vi "Autonomous Independent.vi"() -> ()   [LabVIEW 2014]
doc: "This VI is called when autonomous begins, and will automatically be terminated when autonomous ends. You can carry out timed or sensor driven robot movement independently without needing to return to the caller."
uses:
  <vilib>/Rock Robotics/WPI/RobotDrive/WPI_RobotDriveMecanumDrive_Cartesian.vi
  <vilib>/Rock Robotics/WPI/Solenoid/WPI_SolenoidValue.ctl
  Robot Global Data.vi
  <vilib>/Rock Robotics/WPI/Solenoid/WPI_SolenoidSetEnum.vi
  <vilib>/Rock Robotics/WPI/SafetyOutput/WPI_SafetyOutputConfigMenu.ctl
  navx-mxp_NEW/roborio/labview/navX-MXP Library/navX-MXP IMU.lvlib
  <vilib>/Rock Robotics/Network Tables/SD Read Boolean.vi
  <vilib>/Rock Robotics/Network Tables/SD Read String.vi
  <vilib>/Rock Robotics/Network Tables/SD Write Numeric Array.vi
  <vilib>/Rock Robotics/WPI/RobotDrive/WPI_RobotDriveMecanumDrive_Polar.vi
panel:
  out "MODE: AUTO ZONE":bool
  out "MODE: HPS":bool
  out "AUTO?":bool
  # "EDITED: 3/2/15"
  # "Be sure to right-click and choose Data Operations>>Make Current Value default if you want to save the array values with the VI"
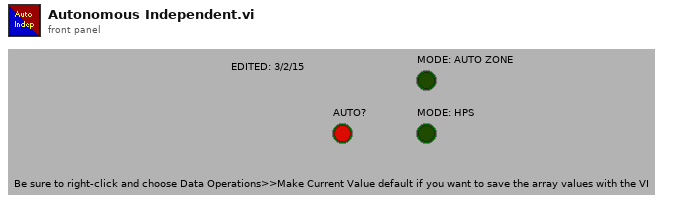
[diagram p1: front panel]
types:
  T1 = typedef "WPI_JoystickDevRef.ctl" = cluster{"Device":T2}
  T2 = typedef "WPI_JoystickDeviceEnum.ctl" = enum16{"USB 0", "USB 1", "USB 2", "USB 3", "USB 4", "USB 5"}
  T3 = typedef "WPI_SafetyOutputConfigMenu.ctl" = enum16{"Enable", "Disable"}
  T4 = typedef "WPI_SolenoidValue.ctl" = enum16{"Off", "On", "Forward", "Reverse"}
  T5 = typedef "navX-MXP IMU.lvlib/navX Device TypeDef.ctl" = cluster{"navX Interface Protocol":T6, "navX Interface Protocol TypeDefs":cluster{"SPIDevRef":T7, "I2CDevRef":T10}, "navX System Information":cluster{"Board Information":T12, "Status":T13, "Offsets":T17}, "navX Common Information":cluster{"Update Rate (4Hz-60Hz)":T18, "refnum name":string, "error":errorcluster}}
  T6 = typedef "navX-MXP IMU.lvlib/navX Interface Protocol.ctl" = enum16{"SPI", "I2C"}
  T7 = typedef "WPI_SPIDevRef.ctl" = cluster{"DevStatus":errorcluster, "Handle":i32, "Controller":T8, "SPI Bus":T9}
  T8 = typedef "FPGA_TypedefDigitalModule.ctl" = enum16{"Controller 1"}
  T9 = typedef "spi_bus.ctl" = enum16{"SPI On-Board, CS0", "SPI On-Board, CS1", "SPI On-Board, CS2", "SPI On-Board, CS3", "SPI MXP", "Invalid"}
  T10 = typedef "WPI_I2CDevRef.ctl" = cluster{"DevStatus":errorcluster, "Controller":T8, "Device Address":u8, "Handle":i32, "I2C Bus":T11}
  T11 = typedef "i2c_bus.ctl" = enum16{"I2C On-Board", "I2C MXP", "Invalid"}
  T12 = typedef "navX-MXP IMU.lvlib/navX Board Information.ctl" = cluster{"WhoAmI (50 | 0x32)":u8, "Board Revision":u8, "Firmware Major Version":u8, "Firmware Minor Version":u8}
  T13 = typedef "navX-MXP IMU.lvlib/navX Status Data.ctl" = cluster{"Update Rate Hz":u8, "Accelerometer Full-Scale Range":u8, "Gyro Full-Scale Range":u16, "NAVX_OP_STATUS":T14, "NAVX_CAL_STATUS":T15, "NAVX_SELFTEST_STATUS":u8, "NAVX_SENSOR_STATUS":T16}
  T14 = typedef "navX-MXP IMU.lvlib/navX NAVX_OP_STATUS.ctl" = u8
  T15 = typedef "navX-MXP IMU.lvlib/navX NAVX_CAL_STATUS.ctl" = u8
  T16 = typedef "navX-MXP IMU.lvlib/navX NAVX_SENSOR_STATUS.ctl" = cluster{"MOVING":bool, "YAW_STABLE":bool, "MAG_DISTURBANCE":bool, "ALTITUDE_VALID":bool, "SEALEVEL_PRESS_SET":bool, "FUSED_HEADING_VALID":bool}
  T17 = typedef "navX-MXP IMU.lvlib/navX Offsets Data.ctl" = cluster{"Yaw":dbl, "Quat W":dbl, "Quat X":dbl, "Quat Y":dbl, "Quat Z":dbl}
  T18 = typedef "navX-MXP IMU.lvlib/navX Update Rate.ctl" = u8
  T19 = cluster{"proportional gain (Kc)":dbl, "integral time (Ti, min)":dbl, "derivative time (Td, min)":dbl}
  T20 = typedef "WPI_RobotDriveDevRef.ctl" = cluster{"DevStatus":errorcluster, "Motors[]":T21[], "Square Inputs":bool, "Max Output":dbl}
  T21 = typedef "WPI_MotorControlDeviceRef.ctl" = cluster{"DeviceStatus":errorcluster, "Type":T22, "PWM":cluster{"Controller":T8, "PWM Channel":T23, "DeadBand":T24}, "CAN":cluster{"Device Number":u8, "Control Mode":T25, "Semaphore":T26, "Max Vout":dbl, "TalonSRX Control Mode":T27}, "Invert":bool, "TransformRef":T28, "InvTransformRef":T28}
  T22 = typedef "WPI_MotorControlType.ctl" = enum16{"PWM", "CAN", "CANTalonSRX"}
  T23 = typedef "FPGA_DIOPWMChannel.ctl" = enum8{"PWM 0", "PWM 1", "PWM 2", "PWM 3", "PWM 4", "PWM 5", "PWM 6", "PWM 7", "PWM 8", "PWM 9", "PWM MXP 0", "PWM MXP 1", "PWM MXP 2", "PWM MXP 3", "PWM MXP 4", "PWM MXP 5", "PWM MXP 6", "PWM MXP 7", "PWM MXP 8", "PWM MXP 9", "Invalid"}
  T24 = typedef "WPI_PWMDeadband.ctl" = cluster{"Name":string, "maxPositivePwm":i32, "minPositivePwm":i32, "centerPwm":i32, "maxNegativePwm":i32, "minNegativePwm":i32, "angularRange":u16}
  T25 = typedef "WPI_CANJaguar_ControlMode.ctl" = enum8{"Percent VBus", "Current", "Speed", "Position", "Voltage"}
  T26 = typedef "Semaphore RefNum" = refnum<k1>
  T27 = typedef "WPI_CANTalonSRX_APIControlMode.ctl" = enum8{"Percent VBus", "Speed", "Position", "Slave", "Unchanged / Invalid"}
  T28 = typedef "WPI_PWMTransform_ConPane.ctl" = refnum<vi>
  T29 = typedef "WPI_SolenoidDevRef.ctl" = cluster{"DevStatus":errorcluster, "Pneumatics Control Module":u8, "Forward Solenoid Channel":T30, "Reverse Solenoid Channel":T30}
  T30 = typedef "WPI_SolenoidChannel.ctl" = enum8{"Solenoid 0", "Solenoid 1", "Solenoid 2", "Solenoid 3", "Solenoid 4", "Solenoid 5", "Solenoid 6", "Solenoid 7", "Invalid"}
  T31 = typedef "WPI_DigitalInputDevRef.ctl" = cluster{"DevStatus":errorcluster, "DIO Channel":T32, "Controller":T8}
  T32 = typedef "FPGA_DIOChannel.ctl" = enum8{"DIO 0", "DIO 1", "DIO 2", "DIO 3", "DIO 4", "DIO 5", "DIO 6", "DIO 7", "DIO 8", "DIO 9", "DIO MXP 0", "DIO MXP 1", "DIO MXP 2", "DIO MXP 3", "DIO MXP 4", "DIO MXP 5", "DIO MXP 6", "DIO MXP 7", "DIO MXP 8", "DIO MXP 9", "DIO MXP 10", "DIO MXP 11", "DIO MXP 12", "DIO MXP 13", "DIO MXP 14", "DIO MXP 15", "Invalid"}
  T33 = cluster{"PID":dbl, "integral time (Ti, min)":dbl, "derivative time (Td, min)":dbl}
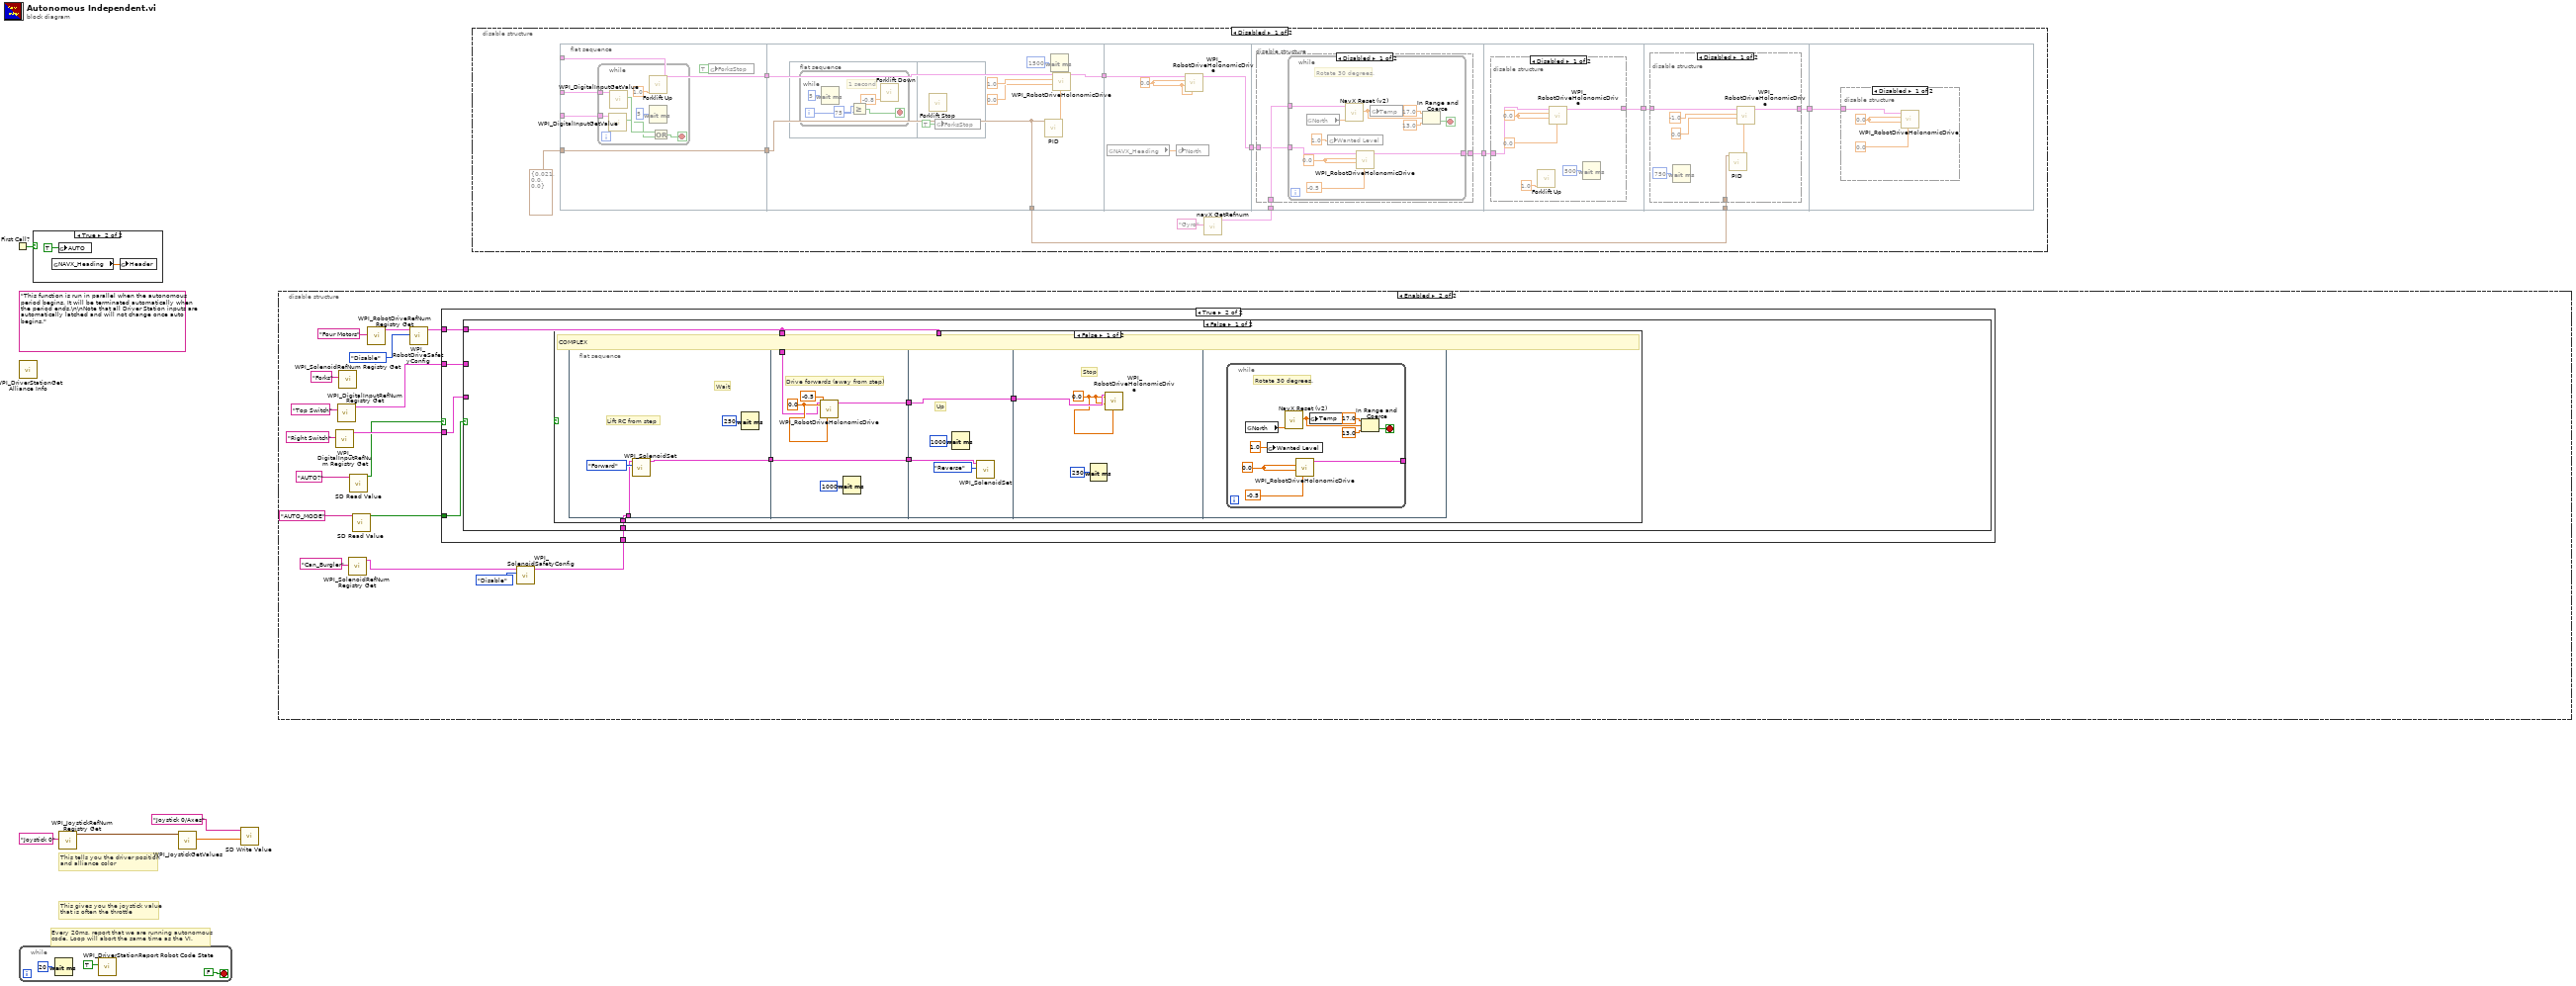
[diagram p0: block diagram]
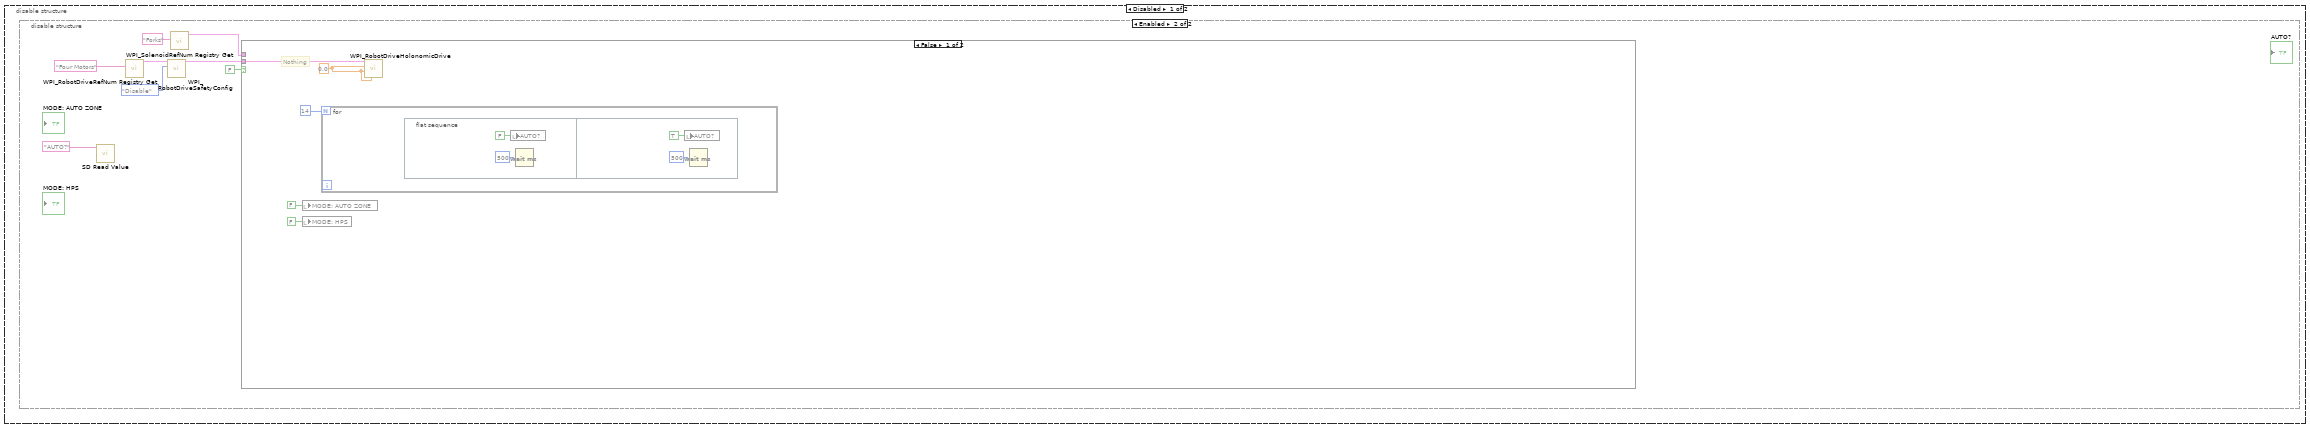
[diagram p7: hidden frame]
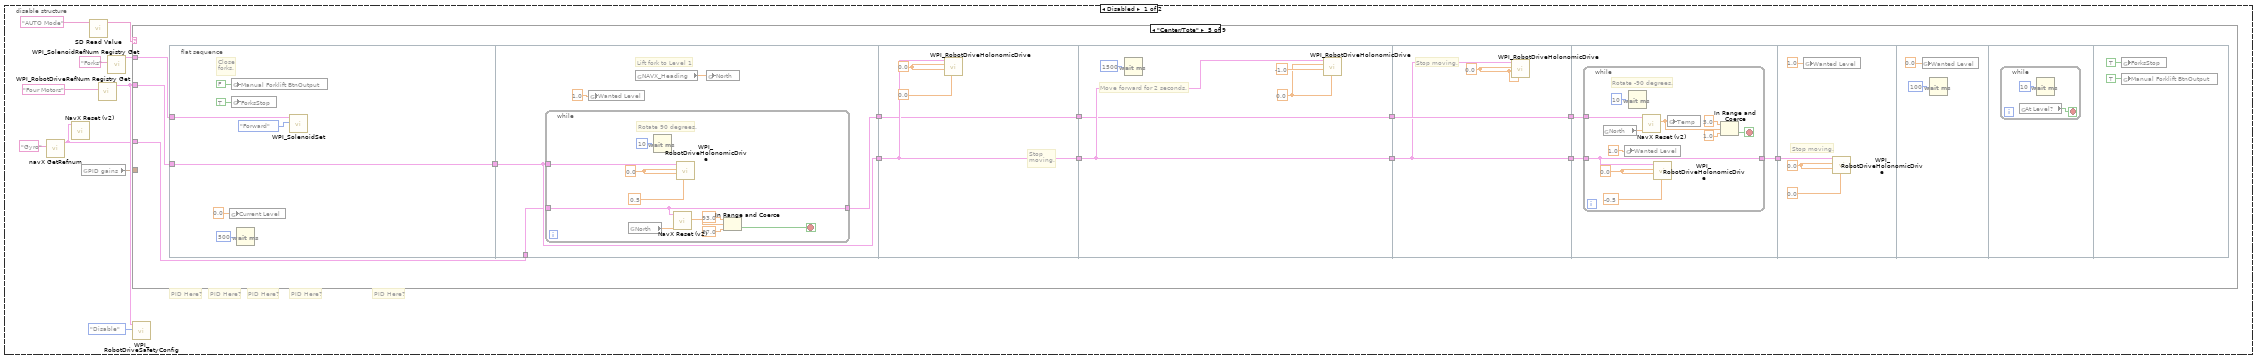
[diagram p8: hidden frame]
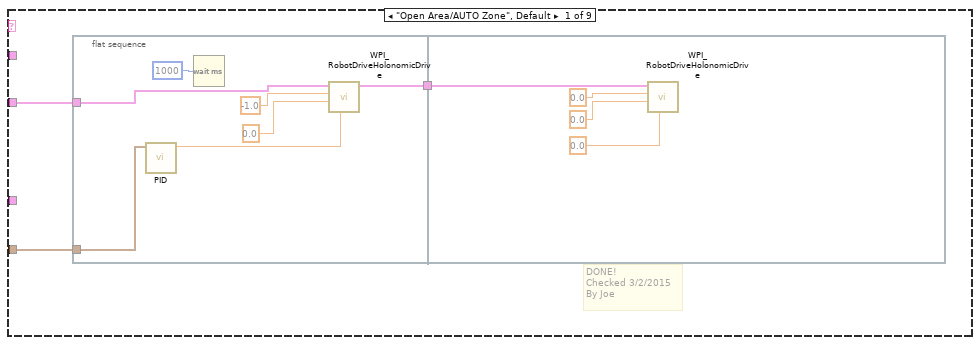
[diagram p9: hidden frame]
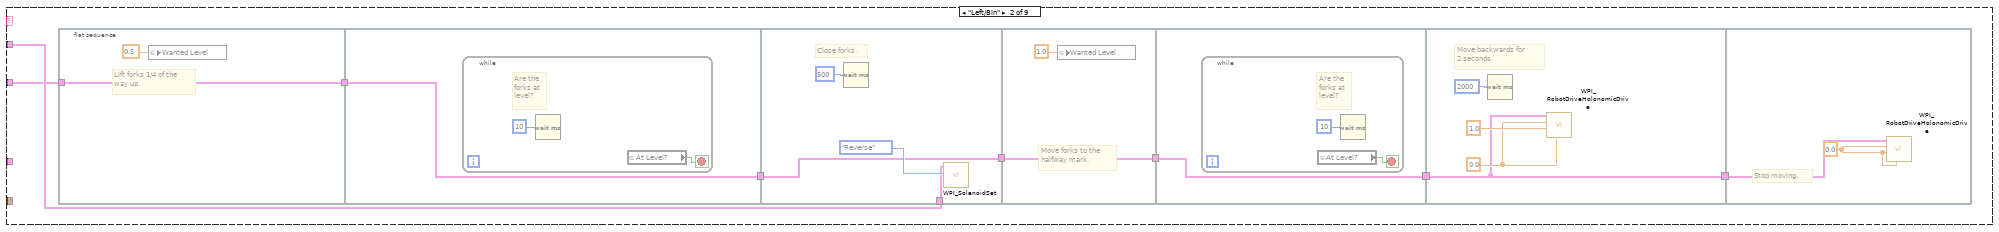
[diagram p10: hidden frame]
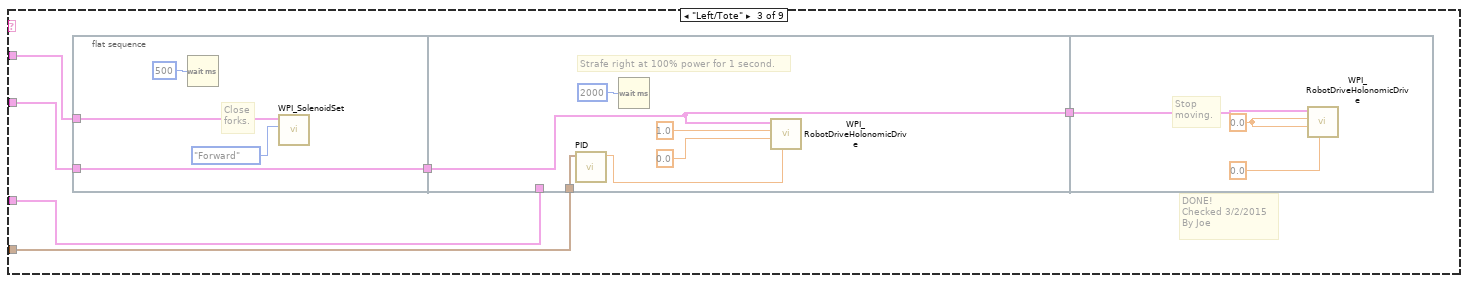
[diagram p11: hidden frame]
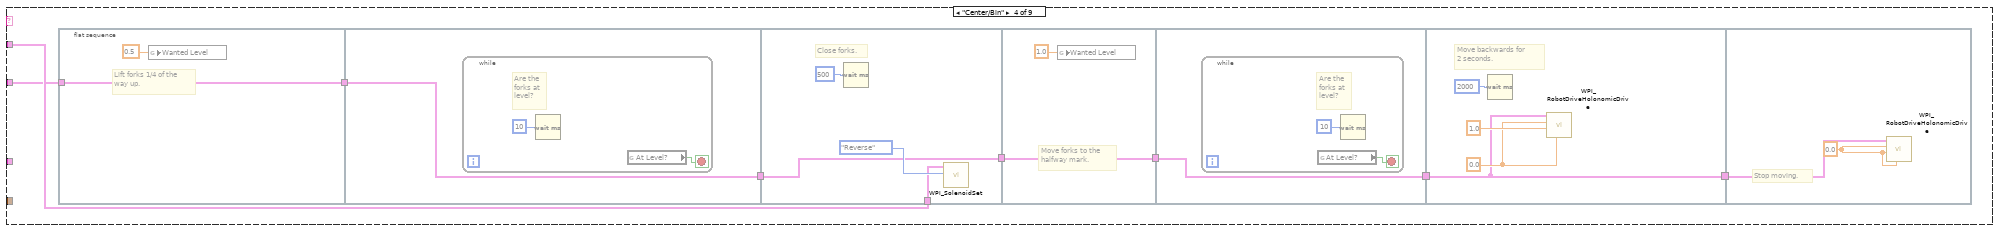
[diagram p12: hidden frame]
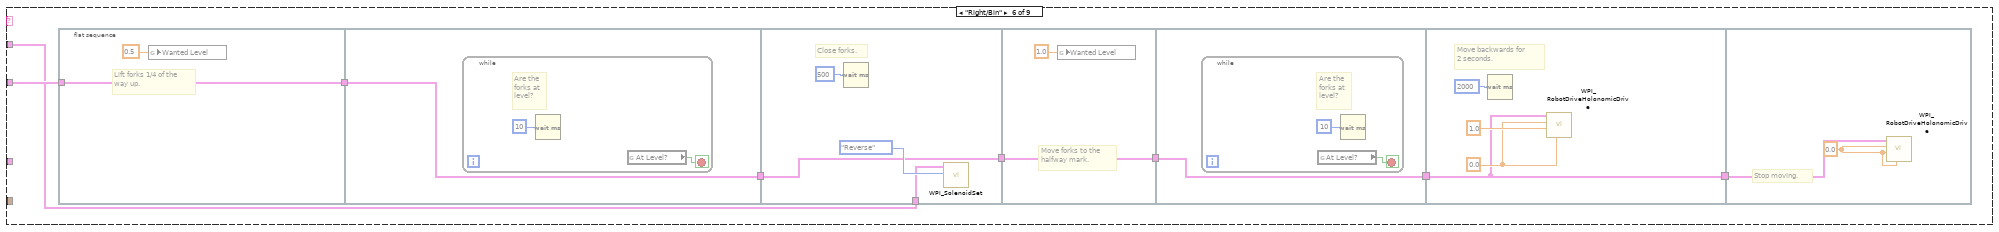
[diagram p13: hidden frame]
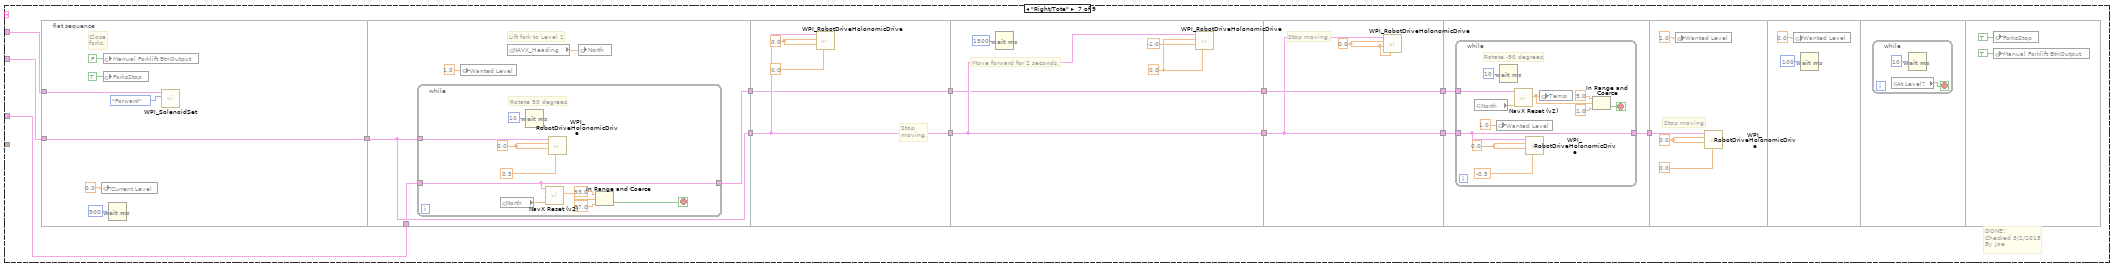
[diagram p14: hidden frame]
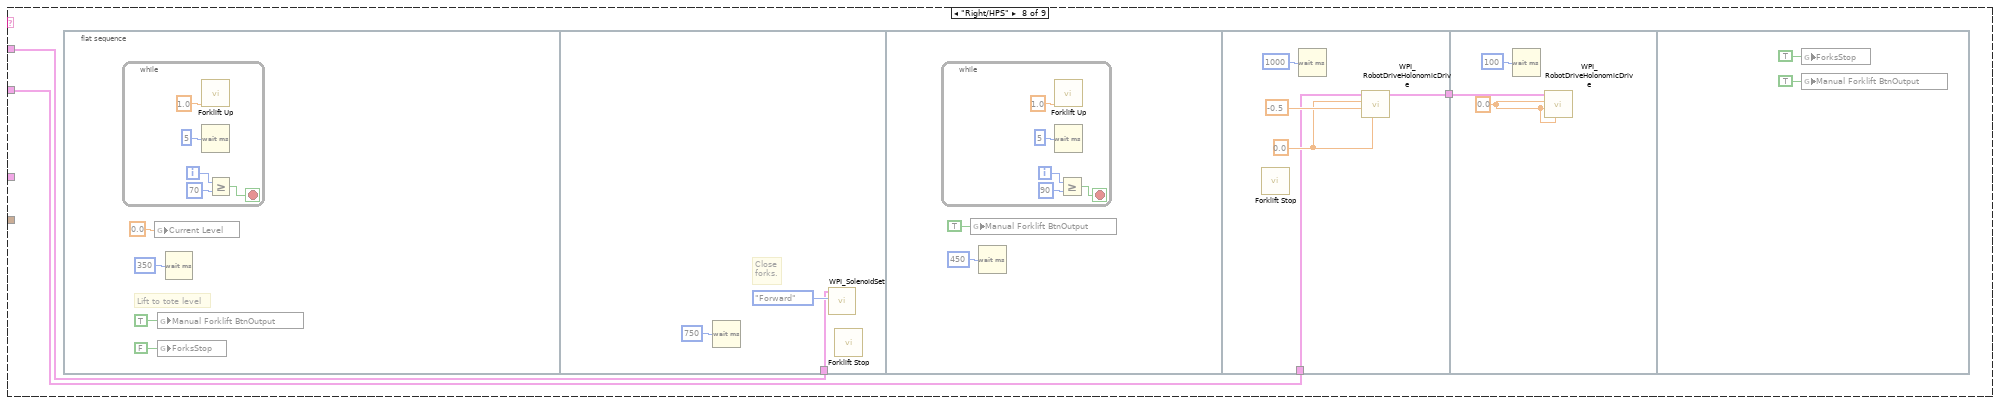
[diagram p15: hidden frame]
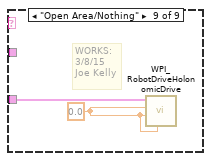
[diagram p16: hidden frame]
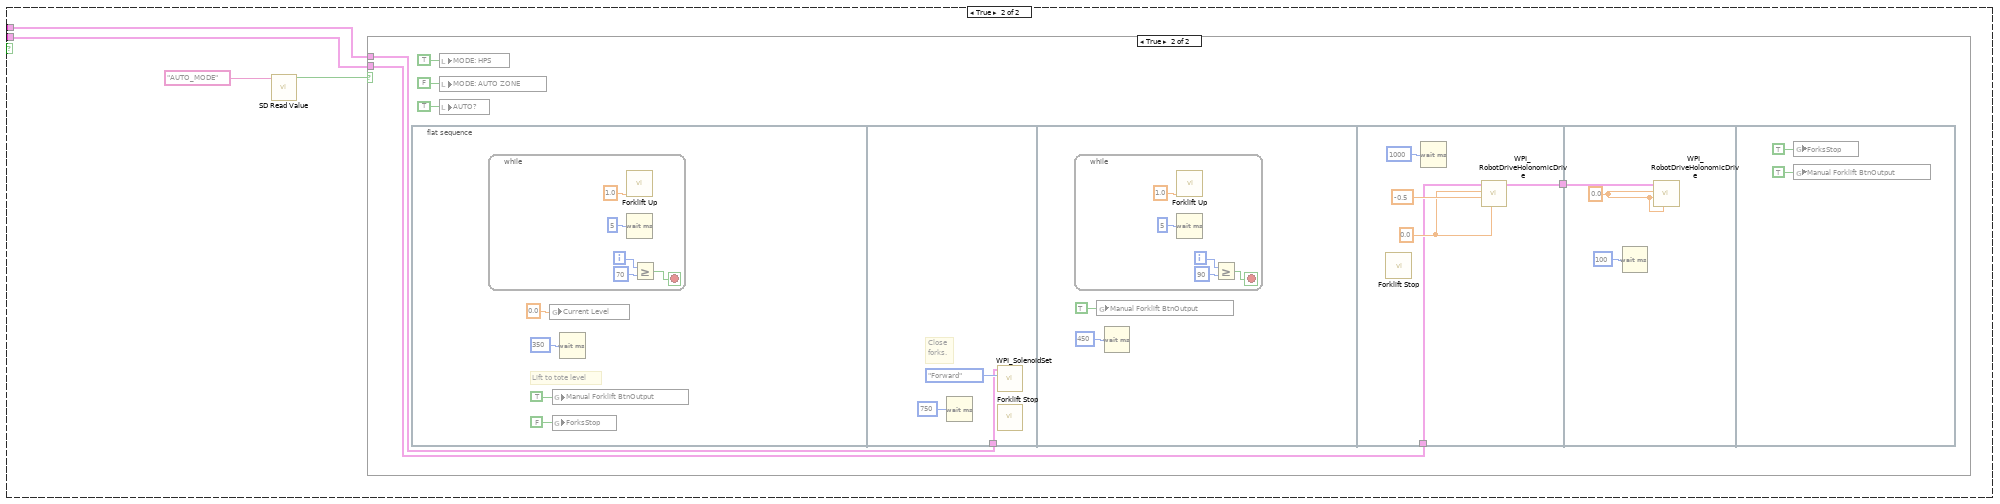
[diagram p17: hidden frame]
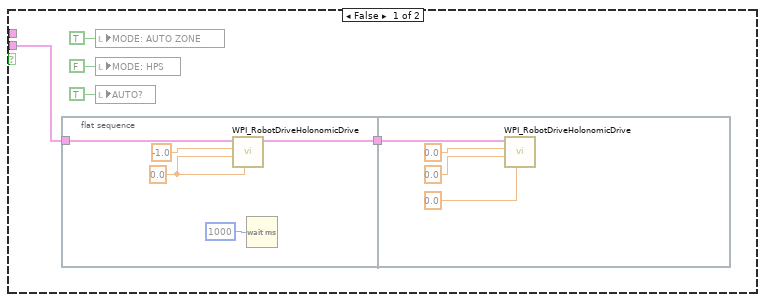
[diagram p18: hidden frame]
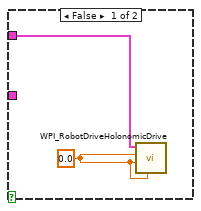
[diagram p19: hidden frame]
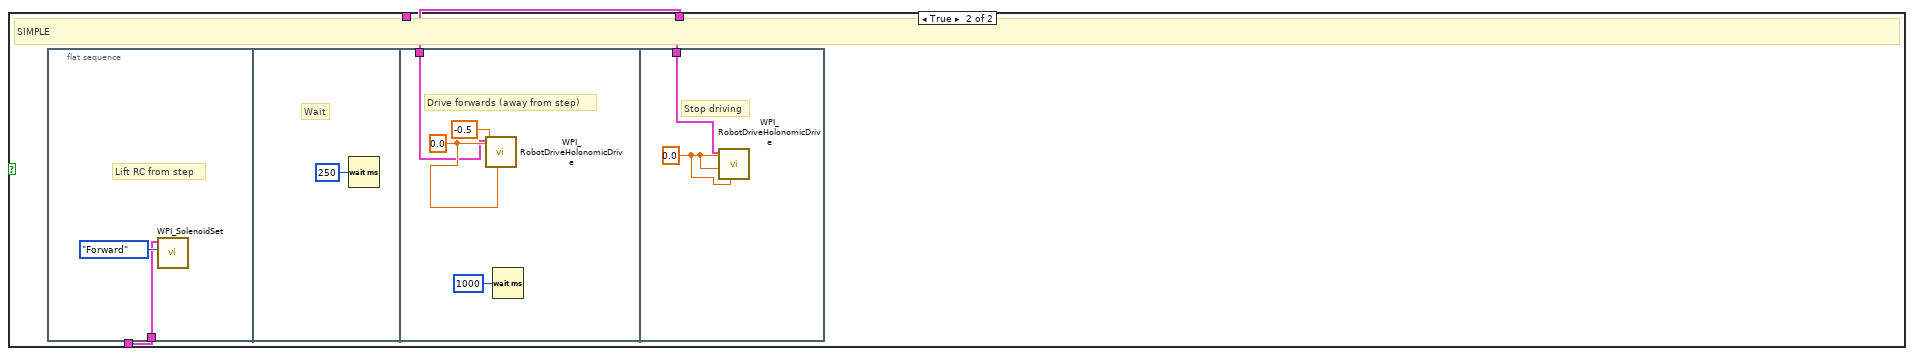
[diagram p20: hidden frame]
diagram:
  (unwired) "This function is run in parallel when the autonomous period begins. It will be terminated automatically when the period ends.\n\nNote that all Driver Station inputs are automatically latched and will not change once auto begins."
  # "Every 20ms, report that we are running autonomous\ncode. Loop will abort the same time as the VI."
  # "This gives you the joystick value\nthat is often the throttle"
  # "This tells you the driver position\nand alliance color"
  n1 = First Call?() -> (First Call?: T/F=w1:bool)
  n2 = call <vilib>:"WPI_DriverStationGet Alliance Info.vi"() -> ()  [unwired: 12 out]
  n3 = while {
    stop <- FALSE stop-if-true
    n4 = Wait (ms)(milliseconds to wait=u32 20) -> ()  [unwired: 1 out]
    n5 = call <vilib>:"WPI_DriverStationReport Robot Code State.vi"("Autonomous"=TRUE) -> ()  [unwired: 10 in, 1 out]
  }
  n6 = case shown="True" w1 {
    frame False {
    }
    frame True {
      n7 = global read "Robot Global Data.vi" "NAVX_Heading"() -> (w10:dbl)
      n8 = global write "Robot Global Data.vi" "AUTO"(TRUE ("AUTO")) -> ()
      n9 = global write "Robot Global Data.vi" "Header"(w10) -> ()
    }
  }
  n10 = call <vilib>:"WPI_JoystickRefNum Registry Get.vi"("refnum name"="Joystick 0") -> ("JoystickDevRef"=w4:T1)  [unwired: 1 in, 9 out]
  n11 = call <vilib>:"WPI_JoystickGetValues.vi"("JoystickDevRef"=w4) -> ("Axes"=w2:dbl[])  [unwired: 6 in, 4 out]
  n12 = call-poly <vilib>:"SD Write Value.vi"("Numeric Array"=w2, "Name"="Joystick 0/Axes") -> ()  [unwired: 8 in, 2 out]
  n13 = disable-structure shown="Enabled" {
    frame Disabled {
      n14 = disable-structure shown="Enabled" {
        frame Disabled {
          # "PID Here?"
          # "PID Here?"
          # "PID Here?"
          # "PID Here?"
          # "PID Here?"
          n15 = call "navX GetRefnum.vi"("refnum name"="Gyro") -> ("navX Device TypeDef"=w13:T5)  [unwired: 9 in, 1 out]
          n16 = call "NavX Reset (v2).vi"("navX Device TypeDef"=w13) -> ()  [unwired: 10 in, 1 out]
          n17 = global read "Robot Global Data.vi" "PID gains"() -> (w12:T19)
          n18 = call-poly <vilib>:"SD Read Value.vi"("Name"="AUTO Mode") -> ("String"=w20:string)  [unwired: 8 in, 2 out]
          n19 = call <vilib>:"WPI_RobotDriveRefNum Registry Get.vi"("refnum name"="Four Motors") -> ("RobotDriveDevRef"=w16:T20)  [unwired: 9 in, 1 out]
          n20 = call <vilib>:"WPI_SolenoidRefNum Registry Get.vi"("refnum name"="Forks") -> ("SolenoidDevRef"=w17:T29)  [unwired: 9 in, 1 out]
          n21 = case shown="\"Center/Tote\"" w20 {
            tunnel: w16 -> [w23 w41 w67 w86 w112 w186 w218 w281 w312]
            tunnel: w17 -> [_ w42 w68 w87 w111 w185 w217 w282 _]
            tunnel: w13 -> [_ _ w65 _ w110 _ w215 _ _]
            tunnel: w12 -> [w21 _ w63 _ _ _ _ _ _]
            frame "Open Area/AUTO Zone", Default {
              # "DONE!\nChecked 3/2/2015\nBy Joe"
              n22 = flat-sequence {
                tunnel: w23 -> [w27]
                tunnel: [w26] -> w22
                tunnel: w21 -> [w24]
                tunnel: w22 -> [w31]
                frame #0 {
                  n23 = call "PID.vi"("PID gains"=w24) -> ("output"=w25:dbl)  [unwired: 10 in]
                  n24 = Wait (ms)(milliseconds to wait=u32 1000) -> ()  [unwired: 1 out]
                  n25 = call-poly <vilib>:"WPI_RobotDriveHolonomicDrive.vi"("Rotation"=w25, "Y"=0.0, "X"=-1.0, "RobotDriveDevRef"=w27) -> ("RobotDriveDevRef"=w26:T20)  [unwired: 5 in, 2 out]
                }
                frame #1 {
                  n26 = call-poly <vilib>:"WPI_RobotDriveHolonomicDrive.vi"("Rotation"=0.0, "Y"=0.0, "X"=0.0, "RobotDriveDevRef"=w31) -> ()  [unwired: 5 in, 3 out]
                }
              }
            }
            frame "Left/Bin" {
              n27 = flat-sequence {
                tunnel: [w43] -> w38
                tunnel: w41 -> [w43]
                tunnel: w38 -> [w45]
                tunnel: [w45] -> w37
                tunnel: w42 -> [w50]
                tunnel: [w49] -> w39
                tunnel: w37 -> [w49]
                tunnel: w39 -> [w53]
                tunnel: [w53] -> w36
                tunnel: w36 -> [w54]
                tunnel: [w54] -> w35
                tunnel: w35 -> [w57]
                tunnel: [w57] -> w40
                tunnel: w40 -> [w61]
                frame #0 {
                  # "Lift forks 1/4 of the\nway up."
                  n28 = global write "Robot Global Data.vi" "Wanted Level"(0.5 ("Wanted Level")) -> ()
                }
                frame #1 {
                  n29 = while {
                    stop <- w47 stop-if-true
                    # "Are the\nforks at\nlevel?"
                    n30 = Wait (ms)(milliseconds to wait=u32 10) -> ()  [unwired: 1 out]
                    n31 = global read "Robot Global Data.vi" "At Level?"() -> (w47:bool)
                  }
                }
                frame #2 {
                  # "Close forks."
                  n32 = Wait (ms)(milliseconds to wait=u32 500) -> ()  [unwired: 1 out]
                  n33 = call-poly <vilib>:"WPI_SolenoidSet.vi"("Value"=WPI_SolenoidValue."Reverse", "SolenoidDevRef"=w50) -> ()  [unwired: 8 in, 2 out]
                }
                frame #3 {
                  # "Move forks to the\nhalfway mark."
                  n34 = global write "Robot Global Data.vi" "Wanted Level"(1.0 ("Wanted Level")) -> ()
                }
                frame #4 {
                  n35 = while {
                    stop <- w56 stop-if-true
                    # "Are the\nforks at\nlevel?"
                    n36 = global read "Robot Global Data.vi" "At Level?"() -> (w56:bool)
                    n37 = Wait (ms)(milliseconds to wait=u32 10) -> ()  [unwired: 1 out]
                  }
                }
                frame #5 {
                  w59 = 0.0 ("X")
                  # "Move backwards for\n2 seconds."
                  n38 = Wait (ms)(milliseconds to wait=u32 2000) -> ()  [unwired: 1 out]
                  n39 = call-poly <vilib>:"WPI_RobotDriveHolonomicDrive.vi"("Rotation"=w59, "Y"=1.0, "X"=w59, "RobotDriveDevRef"=w57) -> ()  [unwired: 5 in, 3 out]
                }
                frame #6 {
                  w62 = 0.0 ("Y")
                  # "Stop moving."
                  n40 = call-poly <vilib>:"WPI_RobotDriveHolonomicDrive.vi"("Rotation"=w62, "Y"=w62, "X"=w62, "RobotDriveDevRef"=w61) -> ()  [unwired: 5 in, 3 out]
                }
              }
            }
            frame "Left/Tote" {
              # "DONE!\nChecked 3/2/2015\nBy Joe"
              n41 = flat-sequence {
                tunnel: w68 -> [w71]
                tunnel: w67 -> [w70]
                tunnel: [w70] -> w64
                tunnel: w64 -> [w76]
                tunnel: [w76] -> w66
                tunnel: w65 -> [_]
                tunnel: w63 -> [w74]
                tunnel: w66 -> [w79]
                frame #0 {
                  # "Close\nforks."
                  n42 = Wait (ms)(milliseconds to wait=u32 500) -> ()  [unwired: 1 out]
                  n43 = call-poly <vilib>:"WPI_SolenoidSet.vi"("Value"=WPI_SolenoidValue."Forward", "SolenoidDevRef"=w71) -> ()  [unwired: 8 in, 2 out]
                }
                frame #1 {
                  # "Strafe right at 100% power for 1 second."
                  n44 = call "PID.vi"("PID gains"=w74) -> ("output"=w73:dbl)  [unwired: 10 in]
                  n45 = Wait (ms)(milliseconds to wait=u32 2000) -> ()  [unwired: 1 out]
                  n46 = call-poly <vilib>:"WPI_RobotDriveHolonomicDrive.vi"("Rotation"=w73, "Y"=0.0, "X"=1.0, "RobotDriveDevRef"=w76) -> ()  [unwired: 5 in, 3 out]
                }
                frame #2 {
                  w80 = 0.0 ("X")
                  # "Stop\nmoving."
                  n47 = call-poly <vilib>:"WPI_RobotDriveHolonomicDrive.vi"("Rotation"=0.0, "Y"=w80, "X"=w80, "RobotDriveDevRef"=w79) -> ()  [unwired: 5 in, 3 out]
                }
              }
            }
            frame "Center/Bin" {
              n48 = flat-sequence {
                tunnel: [w90] -> w85
                tunnel: w86 -> [w90]
                tunnel: w85 -> [w92]
                tunnel: [w92] -> w84
                tunnel: w87 -> [w97]
                tunnel: [w96] -> w89
                tunnel: w84 -> [w96]
                tunnel: w89 -> [w100]
                tunnel: [w100] -> w83
                tunnel: w83 -> [w101]
                tunnel: [w101] -> w82
                tunnel: w82 -> [w104]
                tunnel: [w104] -> w88
                tunnel: w88 -> [w108]
                frame #0 {
                  # "Lift forks 1/4 of the\nway up."
                  n49 = global write "Robot Global Data.vi" "Wanted Level"(0.5 ("Wanted Level")) -> ()
                }
                frame #1 {
                  n50 = while {
                    stop <- w94 stop-if-true
                    # "Are the\nforks at\nlevel?"
                    n51 = Wait (ms)(milliseconds to wait=u32 10) -> ()  [unwired: 1 out]
                    n52 = global read "Robot Global Data.vi" "At Level?"() -> (w94:bool)
                  }
                }
                frame #2 {
                  # "Close forks."
                  n53 = Wait (ms)(milliseconds to wait=u32 500) -> ()  [unwired: 1 out]
                  n54 = call-poly <vilib>:"WPI_SolenoidSet.vi"("Value"=WPI_SolenoidValue."Reverse", "SolenoidDevRef"=w97) -> ()  [unwired: 8 in, 2 out]
                }
                frame #3 {
                  # "Move forks to the\nhalfway mark."
                  n55 = global write "Robot Global Data.vi" "Wanted Level"(1.0 ("Wanted Level")) -> ()
                }
                frame #4 {
                  n56 = while {
                    stop <- w103 stop-if-true
                    # "Are the\nforks at\nlevel?"
                    n57 = global read "Robot Global Data.vi" "At Level?"() -> (w103:bool)
                    n58 = Wait (ms)(milliseconds to wait=u32 10) -> ()  [unwired: 1 out]
                  }
                }
                frame #5 {
                  w106 = 0.0 ("X")
                  # "Move backwards for\n2 seconds."
                  n59 = Wait (ms)(milliseconds to wait=u32 2000) -> ()  [unwired: 1 out]
                  n60 = call-poly <vilib>:"WPI_RobotDriveHolonomicDrive.vi"("Rotation"=w106, "Y"=1.0, "X"=w106, "RobotDriveDevRef"=w104) -> ()  [unwired: 5 in, 3 out]
                }
                frame #6 {
                  w109 = 0.0 ("Y")
                  # "Stop moving."
                  n61 = call-poly <vilib>:"WPI_RobotDriveHolonomicDrive.vi"("Rotation"=w109, "Y"=w109, "X"=w109, "RobotDriveDevRef"=w108) -> ()  [unwired: 5 in, 3 out]
                }
              }
            }
            frame "Center/Tote" {
              n62 = flat-sequence {
                tunnel: w111 -> [w128]
                tunnel: [w123] -> w122
                tunnel: w112 -> [w123]
                tunnel: [w134] -> w121
                tunnel: w122 -> [w134]
                tunnel: w110 -> [w132]
                tunnel: [w131] -> w120
                tunnel: w121 -> [w146]
                tunnel: [w146] -> w119
                tunnel: w120 -> [w145]
                tunnel: [w145] -> w118
                tunnel: w119 -> [w150]
                tunnel: [w150] -> w117
                tunnel: w118 -> [w149]
                tunnel: [w149] -> w116
                tunnel: w117 -> [w154]
                tunnel: w116 -> [w155]
                tunnel: [w155] -> w115
                tunnel: [w154] -> w114
                tunnel: w115 -> [w159]
                tunnel: w114 -> [w158]
                tunnel: [w157] -> w113
                tunnel: w113 -> [w172]
                frame #0 {
                  # "Close\nforks."
                  n63 = global write "Robot Global Data.vi" "Current Level"(0.0 ("Current Level")) -> ()
                  n64 = global write "Robot Global Data.vi" "Manual Forklift BtnOutput"(FALSE ("Manual Forklift BtnOutput")) -> ()
                  n65 = global write "Robot Global Data.vi" "ForksStop"(TRUE ("ForksStop")) -> ()
                  n66 = Wait (ms)(milliseconds to wait=u32 500) -> ()  [unwired: 1 out]
                  n67 = call-poly <vilib>:"WPI_SolenoidSet.vi"("Value"=WPI_SolenoidValue."Forward", "SolenoidDevRef"=w128) -> ()  [unwired: 8 in, 2 out]
                }
                frame #1 {
                  # "Lift fork to Level 1"
                  n68 = while {
                    tunnel: w134 -> [w144]
                    tunnel: w132 -> [w136]
                    tunnel: [w136] -> w131
                    stop <- w140 stop-if-true
                    w141 = 0.0 ("X")
                    # "Rotate 90 degrees."
                    n69 = global read "Robot Global Data.vi" "North"() -> (w135:dbl)
                    n70 = Wait (ms)(milliseconds to wait=u32 10) -> ()  [unwired: 1 out]
                    n71 = call "NavX Reset (v2).vi"("North In"=w135, "navX Device TypeDef"=w136) -> ("Output Angle"=w137:dbl)  [unwired: 9 in]
                    n72 = call-poly <vilib>:"WPI_RobotDriveHolonomicDrive.vi"("Rotation"=0.5, "Y"=w141, "X"=w141, "RobotDriveDevRef"=w144) -> ()  [unwired: 5 in, 3 out]
                    n73 = In Range and Coerce(upper limit=93.0, x=w137, lower limit=87.0) -> (In Range?=w140:bool)  [unwired: 1 out]
                  }
                  n74 = global write "Robot Global Data.vi" "Wanted Level"(1.0 ("Wanted Level")) -> ()
                  n75 = global read "Robot Global Data.vi" "NAVX_Heading"() -> (w130:dbl)
                  n76 = global write "Robot Global Data.vi" "North"(w130) -> ()
                }
                frame #2 {
                  w147 = 0.0 ("X")
                  # "Stop\nmoving."
                  n77 = call-poly <vilib>:"WPI_RobotDriveHolonomicDrive.vi"("Rotation"=0.0, "Y"=w147, "X"=w147, "RobotDriveDevRef"=w146) -> ()  [unwired: 5 in, 3 out]
                }
                frame #3 {
                  w152 = 0.0 ("X")
                  # "Move forward for 2 seconds."
                  n78 = Wait (ms)(milliseconds to wait=u32 1500) -> ()  [unwired: 1 out]
                  n79 = call-poly <vilib>:"WPI_RobotDriveHolonomicDrive.vi"("Rotation"=w152, "Y"=-1.0, "X"=w152, "RobotDriveDevRef"=w150) -> ()  [unwired: 5 in, 3 out]
                }
                frame #4 {
                  w156 = 0.0 ("X")
                  # "Stop moving."
                  n80 = call-poly <vilib>:"WPI_RobotDriveHolonomicDrive.vi"("Rotation"=w156, "Y"=w156, "X"=w156, "RobotDriveDevRef"=w154) -> ()  [unwired: 5 in, 3 out]
                }
                frame #5 {
                  n81 = while {
                    tunnel: w158 -> [w163]
                    tunnel: w159 -> [w164]
                    tunnel: [w163] -> w157
                    stop <- w167 stop-if-true
                    w168 = 0.0 ("X")
                    # "Rotate -90 degrees."
                    n82 = global read "Robot Global Data.vi" "North"() -> (w162:dbl)
                    n83 = global write "Robot Global Data.vi" "Wanted Level"(1.0 ("Wanted Level")) -> ()
                    n84 = Wait (ms)(milliseconds to wait=u32 10) -> ()  [unwired: 1 out]
                    n85 = call "NavX Reset (v2).vi"("North In"=w162, "navX Device TypeDef"=w164) -> ("Output Angle"=w160:dbl)  [unwired: 9 in]
                    n86 = call-poly <vilib>:"WPI_RobotDriveHolonomicDrive.vi"("Rotation"=-0.5, "Y"=w168, "X"=w168, "RobotDriveDevRef"=w163) -> ()  [unwired: 5 in, 3 out]
                    n87 = global write "Robot Global Data.vi" "Temp"(w160) -> ()
                    n88 = In Range and Coerce(upper limit=5.0, x=w160, lower limit=1.0) -> (In Range?=w167:bool)  [unwired: 1 out]
                  }
                }
                frame #6 {
                  w174 = 0.0 ("X")
                  # "Stop moving."
                  n89 = global write "Robot Global Data.vi" "Wanted Level"(1.0 ("Wanted Level")) -> ()
                  n90 = call-poly <vilib>:"WPI_RobotDriveHolonomicDrive.vi"("Rotation"=0.0, "Y"=w174, "X"=w174, "RobotDriveDevRef"=w172) -> ()  [unwired: 5 in, 3 out]
                }
                frame #7 {
                  n91 = global write "Robot Global Data.vi" "Wanted Level"(0.0 ("Wanted Level")) -> ()
                  n92 = Wait (ms)(milliseconds to wait=u32 100) -> ()  [unwired: 1 out]
                }
                frame #8 {
                  n93 = while {
                    stop <- w178 stop-if-true
                    n94 = global read "Robot Global Data.vi" "At Level?"() -> (w178:bool)
                    n95 = Wait (ms)(milliseconds to wait=u32 10) -> ()  [unwired: 1 out]
                  }
                }
                frame #9 {
                  n96 = global write "Robot Global Data.vi" "ForksStop"(TRUE ("ForksStop")) -> ()
                  n97 = global write "Robot Global Data.vi" "Manual Forklift BtnOutput"(TRUE ("Manual Forklift BtnOutput")) -> ()
                }
              }
            }
            frame "Right/Bin" {
              n98 = flat-sequence {
                tunnel: [w189] -> w184
                tunnel: w186 -> [w189]
                tunnel: w184 -> [w191]
                tunnel: [w191] -> w183
                tunnel: w185 -> [w196]
                tunnel: [w195] -> w188
                tunnel: w183 -> [w195]
                tunnel: w188 -> [w199]
                tunnel: [w199] -> w182
                tunnel: w182 -> [w200]
                tunnel: [w200] -> w181
                tunnel: w181 -> [w203]
                tunnel: [w203] -> w187
                tunnel: w187 -> [w207]
                frame #0 {
                  # "Lift forks 1/4 of the\nway up."
                  n99 = global write "Robot Global Data.vi" "Wanted Level"(0.5 ("Wanted Level")) -> ()
                }
                frame #1 {
                  n100 = while {
                    stop <- w192 stop-if-true
                    # "Are the\nforks at\nlevel?"
                    n101 = Wait (ms)(milliseconds to wait=u32 10) -> ()  [unwired: 1 out]
                    n102 = global read "Robot Global Data.vi" "At Level?"() -> (w192:bool)
                  }
                }
                frame #2 {
                  # "Close forks."
                  n103 = Wait (ms)(milliseconds to wait=u32 500) -> ()  [unwired: 1 out]
                  n104 = call-poly <vilib>:"WPI_SolenoidSet.vi"("Value"=WPI_SolenoidValue."Reverse", "SolenoidDevRef"=w196) -> ()  [unwired: 8 in, 2 out]
                }
                frame #3 {
                  # "Move forks to the\nhalfway mark."
                  n105 = global write "Robot Global Data.vi" "Wanted Level"(1.0 ("Wanted Level")) -> ()
                }
                frame #4 {
                  n106 = while {
                    stop <- w202 stop-if-true
                    # "Are the\nforks at\nlevel?"
                    n107 = global read "Robot Global Data.vi" "At Level?"() -> (w202:bool)
                    n108 = Wait (ms)(milliseconds to wait=u32 10) -> ()  [unwired: 1 out]
                  }
                }
                frame #5 {
                  w205 = 0.0 ("X")
                  # "Move backwards for\n2 seconds."
                  n109 = Wait (ms)(milliseconds to wait=u32 2000) -> ()  [unwired: 1 out]
                  n110 = call-poly <vilib>:"WPI_RobotDriveHolonomicDrive.vi"("Rotation"=w205, "Y"=1.0, "X"=w205, "RobotDriveDevRef"=w203) -> ()  [unwired: 5 in, 3 out]
                }
                frame #6 {
                  w208 = 0.0 ("Y")
                  # "Stop moving."
                  n111 = call-poly <vilib>:"WPI_RobotDriveHolonomicDrive.vi"("Rotation"=w208, "Y"=w208, "X"=w208, "RobotDriveDevRef"=w207) -> ()  [unwired: 5 in, 3 out]
                }
              }
            }
            frame "Right/Tote" {
              # "DONE!\nChecked 3/2/2015\nBy Joe"
              n112 = flat-sequence {
                tunnel: w217 -> [w227]
                tunnel: w218 -> [w226]
                tunnel: [w226] -> w221
                tunnel: [w233] -> w220
                tunnel: w221 -> [w233]
                tunnel: w215 -> [w231]
                tunnel: [w230] -> w214
                tunnel: w220 -> [w245]
                tunnel: [w245] -> w219
                tunnel: w214 -> [w244]
                tunnel: [w244] -> w213
                tunnel: w219 -> [w249]
                tunnel: [w249] -> w216
                tunnel: w213 -> [w248]
                tunnel: [w248] -> w212
                tunnel: w216 -> [w253]
                tunnel: w212 -> [w254]
                tunnel: [w254] -> w211
                tunnel: [w253] -> w210
                tunnel: w211 -> [w258]
                tunnel: w210 -> [w257]
                tunnel: [w256] -> w209
                tunnel: w209 -> [w271]
                frame #0 {
                  # "Close\nforks."
                  n113 = global write "Robot Global Data.vi" "Current Level"(0.0 ("Current Level")) -> ()
                  n114 = global write "Robot Global Data.vi" "Manual Forklift BtnOutput"(FALSE ("Manual Forklift BtnOutput")) -> ()
                  n115 = global write "Robot Global Data.vi" "ForksStop"(TRUE ("ForksStop")) -> ()
                  n116 = Wait (ms)(milliseconds to wait=u32 500) -> ()  [unwired: 1 out]
                  n117 = call-poly <vilib>:"WPI_SolenoidSet.vi"("Value"=WPI_SolenoidValue."Forward", "SolenoidDevRef"=w227) -> ()  [unwired: 8 in, 2 out]
                }
                frame #1 {
                  # "Lift fork to Level 1"
                  n118 = while {
                    tunnel: w233 -> [w243]
                    tunnel: w231 -> [w235]
                    tunnel: [w235] -> w230
                    stop <- w239 stop-if-true
                    w240 = 0.0 ("X")
                    # "Rotate 90 degrees."
                    n119 = global read "Robot Global Data.vi" "North"() -> (w234:dbl)
                    n120 = Wait (ms)(milliseconds to wait=u32 10) -> ()  [unwired: 1 out]
                    n121 = call "NavX Reset (v2).vi"("North In"=w234, "navX Device TypeDef"=w235) -> ("Output Angle"=w236:dbl)  [unwired: 9 in]
                    n122 = call-poly <vilib>:"WPI_RobotDriveHolonomicDrive.vi"("Rotation"=0.5, "Y"=w240, "X"=w240, "RobotDriveDevRef"=w243) -> ()  [unwired: 5 in, 3 out]
                    n123 = In Range and Coerce(upper limit=93.0, x=w236, lower limit=87.0) -> (In Range?=w239:bool)  [unwired: 1 out]
                  }
                  n124 = global write "Robot Global Data.vi" "Wanted Level"(1.0 ("Wanted Level")) -> ()
                  n125 = global read "Robot Global Data.vi" "NAVX_Heading"() -> (w229:dbl)
                  n126 = global write "Robot Global Data.vi" "North"(w229) -> ()
                }
                frame #2 {
                  w246 = 0.0 ("X")
                  # "Stop\nmoving."
                  n127 = call-poly <vilib>:"WPI_RobotDriveHolonomicDrive.vi"("Rotation"=0.0, "Y"=w246, "X"=w246, "RobotDriveDevRef"=w245) -> ()  [unwired: 5 in, 3 out]
                }
                frame #3 {
                  w251 = 0.0 ("X")
                  # "Move forward for 2 seconds."
                  n128 = Wait (ms)(milliseconds to wait=u32 1500) -> ()  [unwired: 1 out]
                  n129 = call-poly <vilib>:"WPI_RobotDriveHolonomicDrive.vi"("Rotation"=w251, "Y"=-1.0, "X"=w251, "RobotDriveDevRef"=w249) -> ()  [unwired: 5 in, 3 out]
                }
                frame #4 {
                  w255 = 0.0 ("X")
                  # "Stop moving."
                  n130 = call-poly <vilib>:"WPI_RobotDriveHolonomicDrive.vi"("Rotation"=w255, "Y"=w255, "X"=w255, "RobotDriveDevRef"=w253) -> ()  [unwired: 5 in, 3 out]
                }
                frame #5 {
                  n131 = while {
                    tunnel: w257 -> [w262]
                    tunnel: w258 -> [w263]
                    tunnel: [w262] -> w256
                    stop <- w266 stop-if-true
                    w267 = 0.0 ("X")
                    # "Rotate -90 degrees."
                    n132 = global read "Robot Global Data.vi" "North"() -> (w261:dbl)
                    n133 = global write "Robot Global Data.vi" "Wanted Level"(1.0 ("Wanted Level")) -> ()
                    n134 = Wait (ms)(milliseconds to wait=u32 10) -> ()  [unwired: 1 out]
                    n135 = call "NavX Reset (v2).vi"("North In"=w261, "navX Device TypeDef"=w263) -> ("Output Angle"=w259:dbl)  [unwired: 9 in]
                    n136 = call-poly <vilib>:"WPI_RobotDriveHolonomicDrive.vi"("Rotation"=-0.5, "Y"=w267, "X"=w267, "RobotDriveDevRef"=w262) -> ()  [unwired: 5 in, 3 out]
                    n137 = global write "Robot Global Data.vi" "Temp"(w259) -> ()
                    n138 = In Range and Coerce(upper limit=5.0, x=w259, lower limit=1.0) -> (In Range?=w266:bool)  [unwired: 1 out]
                  }
                }
                frame #6 {
                  w273 = 0.0 ("X")
                  # "Stop moving."
                  n139 = global write "Robot Global Data.vi" "Wanted Level"(1.0 ("Wanted Level")) -> ()
                  n140 = call-poly <vilib>:"WPI_RobotDriveHolonomicDrive.vi"("Rotation"=0.0, "Y"=w273, "X"=w273, "RobotDriveDevRef"=w271) -> ()  [unwired: 5 in, 3 out]
                }
                frame #7 {
                  n141 = global write "Robot Global Data.vi" "Wanted Level"(0.0 ("Wanted Level")) -> ()
                  n142 = Wait (ms)(milliseconds to wait=u32 100) -> ()  [unwired: 1 out]
                }
                frame #8 {
                  n143 = while {
                    stop <- w277 stop-if-true
                    n144 = global read "Robot Global Data.vi" "At Level?"() -> (w277:bool)
                    n145 = Wait (ms)(milliseconds to wait=u32 10) -> ()  [unwired: 1 out]
                  }
                }
                frame #9 {
                  n146 = global write "Robot Global Data.vi" "ForksStop"(TRUE ("ForksStop")) -> ()
                  n147 = global write "Robot Global Data.vi" "Manual Forklift BtnOutput"(TRUE ("Manual Forklift BtnOutput")) -> ()
                }
              }
            }
            frame "Right/HPS" {
              n148 = flat-sequence {
                tunnel: w282 -> [w292]
                tunnel: w281 -> [w304]
                tunnel: [w302] -> w280
                tunnel: w280 -> [w308]
                frame #0 {
                  # "Lift to tote level"
                  n149 = while {
                    i -> [w288]
                    stop <- w289 stop-if-true
                    n150 = call "Forklift Up.vi"("Forklift Up Power"=1.0) -> ()  [unwired: 11 in]
                    n151 = Wait (ms)(milliseconds to wait=u32 5) -> ()  [unwired: 1 out]
                    n152 = Greater Or Equal?(x=w288, y=70) -> (x >= y?=w289:bool)
                  }
                  n153 = global write "Robot Global Data.vi" "Current Level"(0.0 ("Current Level")) -> ()
                  n154 = global write "Robot Global Data.vi" "Manual Forklift BtnOutput"(TRUE ("Manual Forklift BtnOutput")) -> ()
                  n155 = global write "Robot Global Data.vi" "ForksStop"(FALSE ("ForksStop")) -> ()
                  n156 = Wait (ms)(milliseconds to wait=u32 350) -> ()  [unwired: 1 out]
                }
                frame #1 {
                  # "Close\nforks."
                  n157 = Wait (ms)(milliseconds to wait=u32 750) -> ()  [unwired: 1 out]
                  n158 = call-poly <vilib>:"WPI_SolenoidSet.vi"("Value"=WPI_SolenoidValue."Forward", "SolenoidDevRef"=w292) -> ()  [unwired: 8 in, 2 out]
                  n159 = call "Forklift Stop.vi"() -> ()  [unwired: 12 in]
                }
                frame #2 {
                  n160 = while {
                    i -> [w298]
                    stop <- w299 stop-if-true
                    n161 = call "Forklift Up.vi"("Forklift Up Power"=1.0) -> ()  [unwired: 11 in]
                    n162 = Wait (ms)(milliseconds to wait=u32 5) -> ()  [unwired: 1 out]
                    n163 = Greater Or Equal?(x=w298, y=90) -> (x >= y?=w299:bool)
                  }
                  n164 = global write "Robot Global Data.vi" "Manual Forklift BtnOutput"(TRUE ("Manual Forklift BtnOutput")) -> ()
                  n165 = Wait (ms)(milliseconds to wait=u32 450) -> ()  [unwired: 1 out]
                }
                frame #3 {
                  w305 = 0.0 ("X")
                  n166 = call "Forklift Stop.vi"() -> ()  [unwired: 12 in]
                  n167 = Wait (ms)(milliseconds to wait=u32 1000) -> ()  [unwired: 1 out]
                  n168 = call-poly <vilib>:"WPI_RobotDriveHolonomicDrive.vi"("Rotation"=w305, "Y"=-0.5, "X"=w305, "RobotDriveDevRef"=w304) -> ("RobotDriveDevRef"=w302:T20)  [unwired: 5 in, 2 out]
                }
                frame #4 {
                  w309 = 0.0 ("X")
                  n169 = Wait (ms)(milliseconds to wait=u32 100) -> ()  [unwired: 1 out]
                  n170 = call-poly <vilib>:"WPI_RobotDriveHolonomicDrive.vi"("Rotation"=w309, "Y"=w309, "X"=w309, "RobotDriveDevRef"=w308) -> ()  [unwired: 5 in, 3 out]
                }
                frame #5 {
                  n171 = global write "Robot Global Data.vi" "ForksStop"(TRUE ("ForksStop")) -> ()
                  n172 = global write "Robot Global Data.vi" "Manual Forklift BtnOutput"(TRUE ("Manual Forklift BtnOutput")) -> ()
                }
              }
            }
            frame "Open Area/Nothing" {
              w313 = 0.0 ("X")
              # "WORKS:\n3/8/15\nJoe Kelly"
              n173 = call-poly <vilib>:"WPI_RobotDriveHolonomicDrive.vi"("Rotation"=w313, "Y"=w313, "X"=w313, "RobotDriveDevRef"=w312) -> ()  [unwired: 5 in, 3 out]
            }
          }
          n174 = call <vilib>:"WPI_RobotDriveSafetyConfig.vi"("mode"=WPI_SafetyOutputConfigMenu."Disable", "RobotDriveDevRef"=w16) -> ()  [unwired: 8 in, 2 out]
        }
        frame Enabled {
          n175 = call-poly <vilib>:"SD Read Value.vi"("Name"="AUTO?") -> ()  [unwired: 8 in, 3 out]
          n176 = call <vilib>:"WPI_RobotDriveRefNum Registry Get.vi"("refnum name"="Four Motors") -> ("RobotDriveDevRef"=w320:T20)  [unwired: 9 in, 1 out]
          n177 = call <vilib>:"WPI_RobotDriveSafetyConfig.vi"("mode"=WPI_SafetyOutputConfigMenu."Disable", "RobotDriveDevRef"=w320) -> ("RobotDriveDevRef"=w317:T20)  [unwired: 8 in, 1 out]
          n178 = call <vilib>:"WPI_SolenoidRefNum Registry Get.vi"("refnum name"="Forks") -> ("SolenoidDevRef"=w316:T29)  [unwired: 9 in, 1 out]
          n179 = case shown="False" FALSE {
            tunnel: w317 -> [w324 w331]
            tunnel: w316 -> [_ w334]
            frame False {
              w323 = 0.0 ("Magnitude")
              # "Nothing"
              n180 = local write "MODE: AUTO ZONE"(FALSE ("AUTO?")) -> ()
              n181 = local write "MODE: HPS"(FALSE ("AUTO?")) -> ()
              n182 = for {
                N: 14 -> [_]
                n183 = flat-sequence {
                  frame #0 {
                    n184 = local write "AUTO?"(FALSE ("AUTO?")) -> ()
                    n185 = Wait (ms)(milliseconds to wait=u32 500) -> ()  [unwired: 1 out]
                  }
                  frame #1 {
                    n186 = local write "AUTO?"(TRUE ("AUTO?")) -> ()
                    n187 = Wait (ms)(milliseconds to wait=u32 500) -> ()  [unwired: 1 out]
                  }
                }
              }
              n188 = call-poly <vilib>:"WPI_RobotDriveHolonomicDrive.vi"("Rotation"=w323, "Y"=w323, "X"=w323, "RobotDriveDevRef"=w324) -> ()  [unwired: 5 in, 3 out]
            }
            frame True {
              n189 = call-poly <vilib>:"SD Read Value.vi"("Name"="AUTO_MODE") -> ("Boolean"=w333:bool)  [unwired: 8 in, 2 out]
              n190 = case shown="True" w333 {
                tunnel: w334 -> [_ w353]
                tunnel: w331 -> [w338 w349]
                frame False {
                  n191 = flat-sequence {
                    tunnel: [w342] -> w339
                    tunnel: w338 -> [w340]
                    tunnel: w339 -> [w345]
                    frame #0 {
                      w341 = 0.0 ("Y")
                      n192 = call-poly <vilib>:"WPI_RobotDriveHolonomicDrive.vi"("Rotation"=w341, "Y"=w341, "X"=-1.0, "RobotDriveDevRef"=w340) -> ("RobotDriveDevRef"=w342:T20)  [unwired: 5 in, 2 out]
                      n193 = Wait (ms)(milliseconds to wait=u32 1000) -> ()  [unwired: 1 out]
                    }
                    frame #1 {
                      n194 = call-poly <vilib>:"WPI_RobotDriveHolonomicDrive.vi"("Rotation"=0.0, "Y"=0.0, "X"=0.0, "RobotDriveDevRef"=w345) -> ()  [unwired: 5 in, 3 out]
                    }
                  }
                  n195 = local write "MODE: AUTO ZONE"(TRUE ("MODE: AUTO ZONE")) -> ()
                  n196 = local write "MODE: HPS"(FALSE ("MODE: HPS")) -> ()
                  n197 = local write "AUTO?"(TRUE ("AUTO?")) -> ()
                }
                frame True {
                  n198 = flat-sequence {
                    tunnel: w353 -> [w364]
                    tunnel: [w375] -> w354
                    tunnel: w349 -> [w374]
                    tunnel: w354 -> [w380]
                    frame #0 {
                      # "Lift to tote level"
                      n199 = while {
                        i -> [w360]
                        stop <- w361 stop-if-true
                        n200 = call "Forklift Up.vi"("Forklift Up Power"=1.0) -> ()  [unwired: 11 in]
                        n201 = Wait (ms)(milliseconds to wait=u32 5) -> ()  [unwired: 1 out]
                        n202 = Greater Or Equal?(x=w360, y=70) -> (x >= y?=w361:bool)
                      }
                      n203 = global write "Robot Global Data.vi" "Current Level"(0.0 ("Current Level")) -> ()
                      n204 = global write "Robot Global Data.vi" "Manual Forklift BtnOutput"(TRUE ("Manual Forklift BtnOutput")) -> ()
                      n205 = global write "Robot Global Data.vi" "ForksStop"(FALSE ("ForksStop")) -> ()
                      n206 = Wait (ms)(milliseconds to wait=u32 350) -> ()  [unwired: 1 out]
                    }
                    frame #1 {
                      # "Close\nforks."
                      n207 = Wait (ms)(milliseconds to wait=u32 750) -> ()  [unwired: 1 out]
                      n208 = call-poly <vilib>:"WPI_SolenoidSet.vi"("Value"=WPI_SolenoidValue."Forward", "SolenoidDevRef"=w364) -> ()  [unwired: 8 in, 2 out]
                      n209 = call "Forklift Stop.vi"() -> ()  [unwired: 12 in]
                    }
                    frame #2 {
                      n210 = while {
                        i -> [w370]
                        stop <- w371 stop-if-true
                        n211 = call "Forklift Up.vi"("Forklift Up Power"=1.0) -> ()  [unwired: 11 in]
                        n212 = Wait (ms)(milliseconds to wait=u32 5) -> ()  [unwired: 1 out]
                        n213 = Greater Or Equal?(x=w370, y=90) -> (x >= y?=w371:bool)
                      }
                      n214 = global write "Robot Global Data.vi" "Manual Forklift BtnOutput"(TRUE ("Manual Forklift BtnOutput")) -> ()
                      n215 = Wait (ms)(milliseconds to wait=u32 450) -> ()  [unwired: 1 out]
                    }
                    frame #3 {
                      w377 = 0.0 ("X")
                      n216 = call "Forklift Stop.vi"() -> ()  [unwired: 12 in]
                      n217 = Wait (ms)(milliseconds to wait=u32 1000) -> ()  [unwired: 1 out]
                      n218 = call-poly <vilib>:"WPI_RobotDriveHolonomicDrive.vi"("Rotation"=w377, "Y"=-0.5, "X"=w377, "RobotDriveDevRef"=w374) -> ("RobotDriveDevRef"=w375:T20)  [unwired: 5 in, 2 out]
                    }
                    frame #4 {
                      w381 = 0.0 ("X")
                      n219 = Wait (ms)(milliseconds to wait=u32 100) -> ()  [unwired: 1 out]
                      n220 = call-poly <vilib>:"WPI_RobotDriveHolonomicDrive.vi"("Rotation"=w381, "Y"=w381, "X"=w381, "RobotDriveDevRef"=w380) -> ()  [unwired: 5 in, 3 out]
                    }
                    frame #5 {
                      n221 = global write "Robot Global Data.vi" "ForksStop"(TRUE ("ForksStop")) -> ()
                      n222 = global write "Robot Global Data.vi" "Manual Forklift BtnOutput"(TRUE ("Manual Forklift BtnOutput")) -> ()
                    }
                  }
                  n223 = local write "MODE: HPS"(TRUE ("MODE: HPS")) -> ()
                  n224 = local write "MODE: AUTO ZONE"(FALSE ("MODE: HPS")) -> ()
                  n225 = local write "AUTO?"(TRUE ("MODE: HPS")) -> ()
                }
              }
            }
          }
        }
      }
    }
    frame Enabled {
      n226 = call <vilib>:"WPI_DigitalInputRefNum Registry Get.vi"("refnum name"="Right Switch") -> ("DigitalInputDevRef"=w392:T31)  [unwired: 9 in, 1 out]
      n227 = call <vilib>:"WPI_DigitalInputRefNum Registry Get.vi"("refnum name"="Top Switch") -> ("DigitalInputDevRef"=w393:T31)  [unwired: 9 in, 1 out]
      n228 = call <vilib>:"WPI_SolenoidRefNum Registry Get.vi"("refnum name"="Forks") -> ()  [unwired: 9 in, 2 out]
      n229 = call <vilib>:"WPI_SolenoidRefNum Registry Get.vi"("refnum name"="Can_Burgler") -> ("SolenoidDevRef"=w386:T29)  [unwired: 9 in, 1 out]
      n230 = call-poly <vilib>:"SD Read Value.vi"("Name"="AUTO?") -> ("Boolean"=w390:bool)  [unwired: 8 in, 2 out]
      n231 = call-poly <vilib>:"SD Read Value.vi"("Name"="AUTO_MODE") -> ("Boolean"=w388:bool)  [unwired: 8 in, 2 out]
      n232 = call <vilib>:"WPI_RobotDriveRefNum Registry Get.vi"("refnum name"="Four Motors") -> ("RobotDriveDevRef"=w398:T20)  [unwired: 9 in, 1 out]
      n233 = call <vilib>:"WPI_RobotDriveSafetyConfig.vi"("mode"=WPI_SafetyOutputConfigMenu."Disable", "RobotDriveDevRef"=w398) -> ("RobotDriveDevRef"=w396:T20)  [unwired: 8 in, 1 out]
      n234 = call <vilib>:"WPI_SolenoidSafetyConfig.vi"("mode"=WPI_SafetyOutputConfigMenu."Disable", "SolenoidDevRef"=w386) -> ("SolenoidDevRef 2"=w385:T29)  [unwired: 8 in, 1 out]
      n235 = case shown="True" w390 {
        tunnel: w396 -> [w401 w407]
        tunnel: w393 -> [_ w406]
        tunnel: w392 -> [_ w405]
        tunnel: w388 -> [_ w404]
        tunnel: w385 -> [_ w403]
        frame False {
          w402 = 0.0 ("Y")
          n236 = call-poly <vilib>:"WPI_RobotDriveHolonomicDrive.vi"("Rotation"=w402, "Y"=w402, "X"=w402, "RobotDriveDevRef"=w401) -> ()  [unwired: 5 in, 3 out]
        }
        frame True {
          n237 = case shown="False" w404 {
            tunnel: w407 -> [w408 w453]
            tunnel: w406 -> [_ _]
            tunnel: w405 -> [_ _]
            tunnel: w403 -> [w409 _]
            frame False {
              n238 = case shown="False" {
                selector: _ -> [_ _]
                tunnel: w408 -> [_ w443]
                tunnel: w409 -> [w415 w442]
                tunnel: w408 -> [w414 _]
                frame False {
                  # "COMPLEX"
                  n239 = flat-sequence {
                    tunnel: [w418] -> w412
                    tunnel: w415 -> [w416]
                    tunnel: w414 -> [w423]
                    tunnel: [w422] -> w413
                    tunnel: w412 -> [w421]
                    tunnel: [w421] -> w411
                    tunnel: w413 -> [w426]
                    tunnel: w411 -> [w428]
                    tunnel: [w426] -> w410
                    tunnel: w410 -> [w432]
                    frame #0 {
                      # "Lift RC from step"
                      # "Wait"
                      n240 = call-poly <vilib>:"WPI_SolenoidSet.vi"("Value"=WPI_SolenoidValue."Forward", "SolenoidDevRef"=w416) -> ("SolenoidDevRef"=w418:T29)  [unwired: 8 in, 1 out]
                      n241 = Wait (ms)(milliseconds to wait=u32 250) -> ()  [unwired: 1 out]
                    }
                    frame #1 {
                      w424 = 0.0 ("X")
                      # "Drive forwards (away from step)"
                      n242 = call-poly <vilib>:"WPI_RobotDriveHolonomicDrive.vi"("Rotation"=w424, "Y"=-0.5, "X"=w424, "RobotDriveDevRef"=w423) -> ("RobotDriveDevRef"=w422:T20)  [unwired: 5 in, 2 out]
                      n243 = Wait (ms)(milliseconds to wait=u32 1000) -> ()  [unwired: 1 out]
                    }
                    frame #2 {
                      # "Up"
                      n244 = Wait (ms)(milliseconds to wait=u32 1000) -> ()  [unwired: 1 out]
                      n245 = call-poly <vilib>:"WPI_SolenoidSet.vi"("Value"=WPI_SolenoidValue."Reverse", "SolenoidDevRef"=w428) -> ()  [unwired: 8 in, 2 out]
                    }
                    frame #3 {
                      w431 = 0.0 ("X")
                      # "Stop"
                      n246 = Wait (ms)(milliseconds to wait=u32 250) -> ()  [unwired: 1 out]
                      n247 = call-poly <vilib>:"WPI_RobotDriveHolonomicDrive.vi"("Rotation"=w431, "Y"=w431, "X"=w431, "RobotDriveDevRef"=w432) -> ()  [unwired: 5 in, 3 out]
                    }
                    frame #4 {
                      n248 = while {
                        tunnel: [w433] -> _
                        stop <- w439 stop-if-true
                        w440 = 0.0 ("X")
                        # "Rotate 30 degrees."
                        n249 = global read "Robot Global Data.vi" "North"() -> (w436:dbl)
                        n250 = global write "Robot Global Data.vi" "Wanted Level"(1.0 ("Wanted Level")) -> ()
                        n251 = call "NavX Reset (v2).vi"("North In"=w436) -> ("Output Angle"=w434:dbl)  [unwired: 10 in]
                        n252 = call-poly <vilib>:"WPI_RobotDriveHolonomicDrive.vi"("Rotation"=-0.5, "Direction"=w440, "Magnitude"=w440) -> ("RobotDriveDevRef"=w433:T20)  [unwired: 6 in, 2 out]
                        n253 = global write "Robot Global Data.vi" "Temp"(w434) -> ()
                        n254 = In Range and Coerce(upper limit=17.0, x=w434, lower limit=13.0) -> (In Range?=w439:bool)  [unwired: 1 out]
                      }
                    }
                  }
                }
                frame True {
                  # "SIMPLE"
                  n255 = flat-sequence {
                    tunnel: w442 -> [w444]
                    tunnel: w443 -> [w447]
                    tunnel: w443 -> [w451]
                    frame #0 {
                      # "Lift RC from step"
                      n256 = call-poly <vilib>:"WPI_SolenoidSet.vi"("Value"=WPI_SolenoidValue."Forward", "SolenoidDevRef"=w444) -> ()  [unwired: 8 in, 2 out]
                    }
                    frame #1 {
                      # "Wait"
                      n257 = Wait (ms)(milliseconds to wait=u32 250) -> ()  [unwired: 1 out]
                    }
                    frame #2 {
                      w448 = 0.0 ("X")
                      # "Drive forwards (away from step)"
                      n258 = call-poly <vilib>:"WPI_RobotDriveHolonomicDrive.vi"("Rotation"=w448, "Y"=-0.5, "X"=w448, "RobotDriveDevRef"=w447) -> ()  [unwired: 5 in, 3 out]
                      n259 = Wait (ms)(milliseconds to wait=u32 1000) -> ()  [unwired: 1 out]
                    }
                    frame #3 {
                      w452 = 0.0 ("X")
                      # "Stop driving"
                      n260 = call-poly <vilib>:"WPI_RobotDriveHolonomicDrive.vi"("Rotation"=w452, "Y"=w452, "X"=w452, "RobotDriveDevRef"=w451) -> ()  [unwired: 5 in, 3 out]
                    }
                  }
                }
              }
            }
            frame True {
              # "Strafe LEFT"
              n261 = flat-sequence {
                tunnel: [w457] -> w454
                tunnel: w453 -> [w455]
                tunnel: w454 -> [w460]
                frame #0 {
                  w456 = 0.0 ("Y")
                  n262 = call-poly <vilib>:"WPI_RobotDriveHolonomicDrive.vi"("Rotation"=w456, "Y"=w456, "X"=-1.0, "RobotDriveDevRef"=w455) -> ("RobotDriveDevRef"=w457:T20)  [unwired: 5 in, 2 out]
                  n263 = Wait (ms)(milliseconds to wait=u32 1000) -> ()  [unwired: 1 out]
                }
                frame #1 {
                  n264 = call-poly <vilib>:"WPI_RobotDriveHolonomicDrive.vi"("Rotation"=0.0, "Y"=0.0, "X"=0.0, "RobotDriveDevRef"=w460) -> ()  [unwired: 5 in, 3 out]
                }
              }
            }
          }
        }
      }
    }
  }
  n265 = disable-structure shown="Disabled" {
    frame Disabled {
      n266 = flat-sequence {
        tunnel: T33 {"PID"=0.021, "integral time (Ti, min)"=0.0, "derivative time (Td, min)"=0.0} ("PID gains") -> [w481]
        tunnel: [w482] -> w464
        tunnel: [w482] -> w477
        tunnel: [w481] -> w476
        tunnel: [w480] -> w466
        tunnel: [w479] -> w467
        tunnel: [w495] -> w475
        tunnel: w477 -> [w496]
        tunnel: w476 -> [w490]
        tunnel: [w490] -> w470
        tunnel: w475 -> [w506]
        tunnel: [w504] -> w474
        tunnel: w469 -> [w509]
        tunnel: w474 -> [w508]
        tunnel: [w507] -> w473
        tunnel: w473 -> [w525]
        tunnel: [w524] -> w472
        tunnel: w470 -> [w534]
        tunnel: w472 -> [w533]
        tunnel: [w532] -> w471
        tunnel: w471 -> [w542]
        frame #0 {
          n267 = while {
            tunnel: w480 -> [w486]
            tunnel: w479 -> [w485]
            stop <- w487 stop-if-true
            n268 = call <vilib>:"WPI_DigitalInputGetValue.vi"("DigitalInputDevRef"=w485) -> ("Value"=w483:bool)  [unwired: 8 in, 2 out]
            n269 = call <vilib>:"WPI_DigitalInputGetValue.vi"("DigitalInputDevRef"=w486) -> ("Value"=w484:bool)  [unwired: 8 in, 2 out]
            n270 = call "Forklift Up.vi"("Forklift Up Power"=1.0) -> ()  [unwired: 11 in]
            n271 = Wait (ms)(milliseconds to wait=u32 5) -> ()  [unwired: 1 out]
            n272 = Or(x=w484, y=w483) -> (x .or. y?=w487:bool)
          }
          n273 = global write "Robot Global Data.vi" "ForksStop"(TRUE ("AUTO")) -> ()
        }
        frame #1 {
          n274 = flat-sequence {
            frame #0 {
              n275 = while {
                i -> [w501]
                stop <- w498 stop-if-true
                # "1 second"
                n276 = Wait (ms)(milliseconds to wait=u32 5) -> ()  [unwired: 1 out]
                n277 = Greater Or Equal?(x=w501, y=75) -> (x >= y?=w498:bool)
                n278 = call "Forklift Down.vi"("Forklift Down Speed"=-0.8) -> ()  [unwired: 11 in]
              }
            }
            frame #1 {
              n279 = call "Forklift Stop.vi"() -> ()  [unwired: 12 in]
              n280 = global write "Robot Global Data.vi" "ForksStop"(TRUE ("ForksStop")) -> ()
            }
          }
          n281 = call "PID.vi"("PID gains"=w490) -> ("output"=w492:dbl)  [unwired: 10 in]
          n282 = Wait (ms)(milliseconds to wait=u32 1500) -> ()  [unwired: 1 out]
          n283 = call-poly <vilib>:"WPI_RobotDriveHolonomicDrive.vi"("Rotation"=w492, "Y"=0.0, "X"=1.0, "RobotDriveDevRef"=w496) -> ("RobotDriveDevRef"=w495:T20)  [unwired: 5 in, 2 out]
        }
        frame #2 {
          w505 = 0.0 ("Y")
          n284 = global read "Robot Global Data.vi" "NAVX_Heading"() -> (w503:dbl)
          n285 = global write "Robot Global Data.vi" "North"(w503) -> ()
          n286 = call-poly <vilib>:"WPI_RobotDriveHolonomicDrive.vi"("Rotation"=w505, "Y"=w505, "X"=w505, "RobotDriveDevRef"=w506) -> ("RobotDriveDevRef"=w504:T20)  [unwired: 5 in, 2 out]
        }
        frame #3 {
          n287 = disable-structure shown="Disabled" {
            disable-tunnel: w509 -> [w512 _]
            disable-tunnel: w508 -> [w511 _]
            disable-tunnel: [w510 _] -> w507
            frame Disabled {
              n288 = while {
                tunnel: w511 -> [w517]
                tunnel: w512 -> [w518]
                tunnel: [w513] -> w510
                stop <- w521 stop-if-true
                w522 = 0.0 ("X")
                # "Rotate 30 degrees."
                n289 = global read "Robot Global Data.vi" "North"() -> (w516:dbl)
                n290 = global write "Robot Global Data.vi" "Wanted Level"(1.0 ("Wanted Level")) -> ()
                n291 = call "NavX Reset (v2).vi"("North In"=w516, "navX Device TypeDef"=w518) -> ("Output Angle"=w514:dbl)  [unwired: 9 in]
                n292 = call-poly <vilib>:"WPI_RobotDriveHolonomicDrive.vi"("Rotation"=-0.5, "Y"=w522, "X"=w522, "RobotDriveDevRef"=w517) -> ("RobotDriveDevRef"=w513:T20)  [unwired: 5 in, 2 out]
                n293 = global write "Robot Global Data.vi" "Temp"(w514) -> ()
                n294 = In Range and Coerce(upper limit=17.0, x=w514, lower limit=13.0) -> (In Range?=w521:bool)  [unwired: 1 out]
              }
            }
            frame Enabled {
            }
          }
        }
        frame #4 {
          n295 = disable-structure shown="Disabled" {
            disable-tunnel: w525 -> [w529 _]
            disable-tunnel: [w526 _] -> w524
            frame Disabled {
              w531 = 0.0 ("X")
              n296 = call "Forklift Up.vi"("Forklift Up Power"=1.0) -> ()  [unwired: 11 in]
              n297 = call-poly <vilib>:"WPI_RobotDriveHolonomicDrive.vi"("Rotation"=0.0, "Y"=w531, "X"=w531, "RobotDriveDevRef"=w529) -> ("RobotDriveDevRef"=w526:T20)  [unwired: 5 in, 2 out]
              n298 = Wait (ms)(milliseconds to wait=u32 500) -> ()  [unwired: 1 out]
            }
            frame Enabled {
            }
          }
        }
        frame #5 {
          n299 = disable-structure shown="Disabled" {
            disable-tunnel: w534 -> [w538 _]
            disable-tunnel: w533 -> [w536 _]
            disable-tunnel: [w535 _] -> w532
            frame Disabled {
              n300 = Wait (ms)(milliseconds to wait=u32 750) -> ()  [unwired: 1 out]
              n301 = call "PID.vi"("PID gains"=w538) -> ("output"=w540:dbl)  [unwired: 10 in]
              n302 = call-poly <vilib>:"WPI_RobotDriveHolonomicDrive.vi"("Rotation"=w540, "Y"=0.0, "X"=-1.0, "RobotDriveDevRef"=w536) -> ("RobotDriveDevRef"=w535:T20)  [unwired: 5 in, 2 out]
            }
            frame Enabled {
            }
          }
        }
        frame #6 {
          n303 = disable-structure shown="Disabled" {
            disable-tunnel: w542 -> [w543 _]
            frame Disabled {
              w545 = 0.0 ("X")
              n304 = call-poly <vilib>:"WPI_RobotDriveHolonomicDrive.vi"("Rotation"=0.0, "Y"=w545, "X"=w545, "RobotDriveDevRef"=w543) -> ()  [unwired: 5 in, 3 out]
            }
            frame Enabled {
            }
          }
        }
      }
      n305 = call "navX GetRefnum.vi"("refnum name"="Gyro") -> ("navX Device TypeDef"=w469:T5)  [unwired: 9 in, 1 out]
    }
    frame Enabled {
    }
  }
